vi "Simple RT Add-setup.vi"(7 "test case ID":string) -> (1 "y":dbl, 2 "x":dbl)   [LabVIEW 2018]
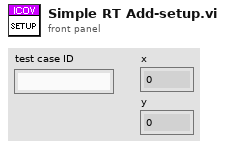
[diagram p1: front panel]
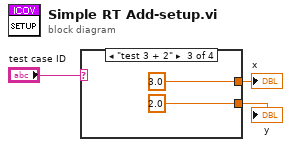
[diagram p0: block diagram]
diagram:
  n1 = case shown="\"test 3 + 2\"" "test case ID" {
    tunnel: [_ _ 3.0 ("x") _] -> w2
    tunnel: [_ _ 2.0 ("y") _] -> w1
    frame "testcaseID1" {
    }
    frame "testcaseID2" {
    }
    frame "test 3 + 2" {
    }
    frame Default {
    }
  }
  "x" <- w2
  "y" <- w1
